vi "Cluster Replacement.vi"() -> ()   [LabVIEW 2020]
panel:
  out "array":dbl[](array[numeric])
  out "Array":dbl[](array[numeric])
  in  "New Element":dbl
  out "Numeric":dbl
  in  "Independent Variable":u16(ring) items=["A", "B"]
  in  "B":dbl
  in  "A":dbl
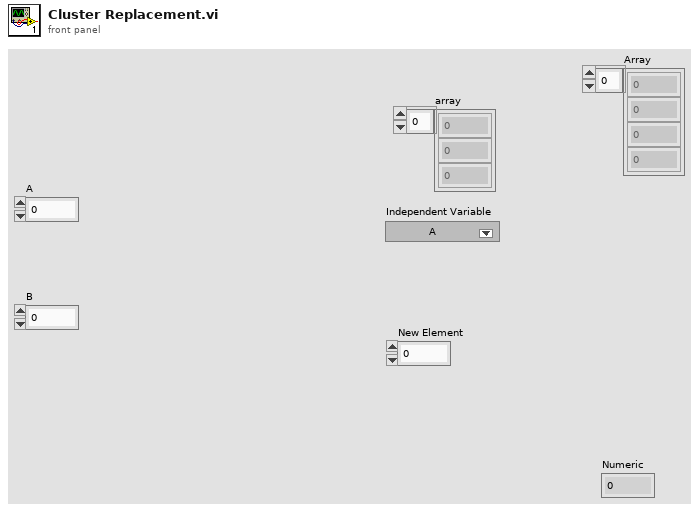
[diagram p1: front panel]
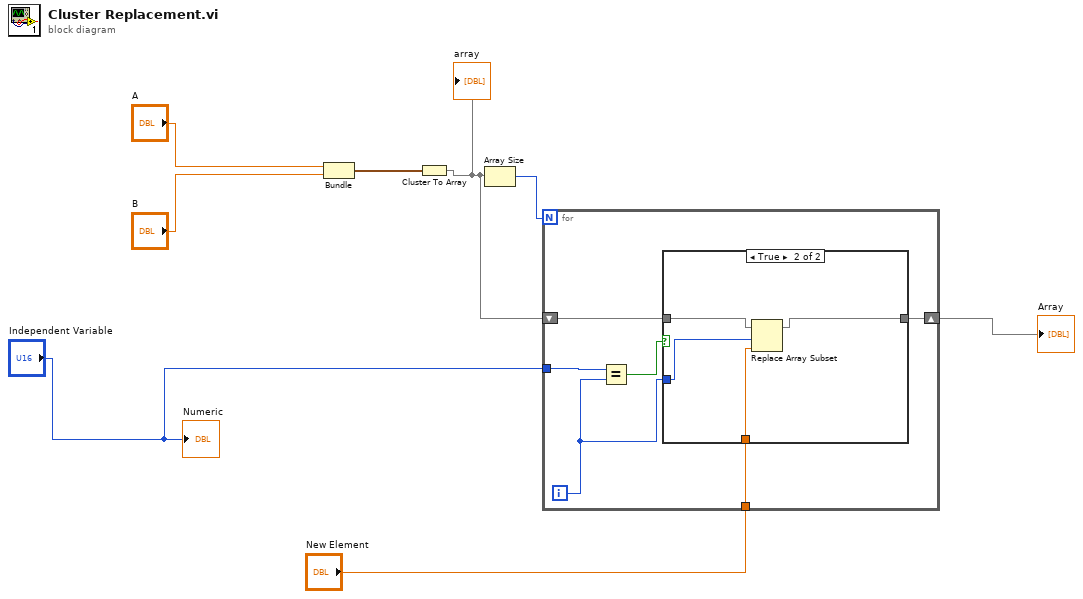
[diagram p0: block diagram]
diagram:
  n1 = Bundle("A"="A", "B"="B") -> (w6:cluster{"A":dbl, "B":dbl})  [unwired: 1 in]
  n2 = Cluster To Array(cluster=w6) -> (array=w4:dbl[])
  "array" <- w4
  n3 = Array Size(array=w4) -> (size(s)=w5:i32)
  n4 = for {
    N: w5 -> [_]
    shift-right: [w14] -> w1
    shift-left: w4 -> [w13]
    tunnel: "Independent Variable" -> [w11]
    tunnel: "New Element" -> [w9]
    i -> [w10]
    n5 = Equal?(x=w11, y=w10) -> (x = y?=w12:bool)
    n6 = case shown="True" w12 {
      tunnel: w13 -> [w15 w17]
      tunnel: [w15 w16] -> w14
      tunnel: w10 -> [_ w19]
      tunnel: w9 -> [_ w18]
      frame False {
      }
      frame True {
        n7 = Replace Array Subset(array=w17, new element=w18, index=w19) -> (w16:dbl[])
      }
    }
  }
  "Array" <- w1
  "Numeric" <- "Independent Variable"
